vi "Teleop.vi"(10 "Match Info":T1={"Autonomous Elapsed Seconds"=0.0, "TeleOp Elapsed Seconds"=0.0, "Disabled Elapsed Seconds"=0.0, "Visited Autonomous"=FALSE, "Visited TeleOp"=FALSE, "Visited Disabled"=FALSE, "Autonomous Settings"={"Autonomous Style"=enum."Independent", "VI Refnum"=refnum}}, 11 "Call Context":T2) -> ()   [LabVIEW 2014]
doc: "This VI is called for each TeleOp packet received from the DS where the robot is not disabled. It is often used to read from the joysticks and update I/O or to update setpoints for timed control loops. It should complete and return within 20 milliseconds or it may miss DS packets."
uses:
  <vilib>/Rock Robotics/WPI/DriverStation/WPI_DriverStationDerivedRobotMode.ctl
  <vilib>/Rock Robotics/WPI/DriverStation/WPI_DriverStationMatch Info.ctl
  <vilib>/Rock Robotics/WPI/Joystick/WPI_JoystickGetSetRefNum.vi
  Robot Global Data.vi
panel:
  out "Loop Time":cluster{"X":dbl[], "Y":dbl[]}(graph)
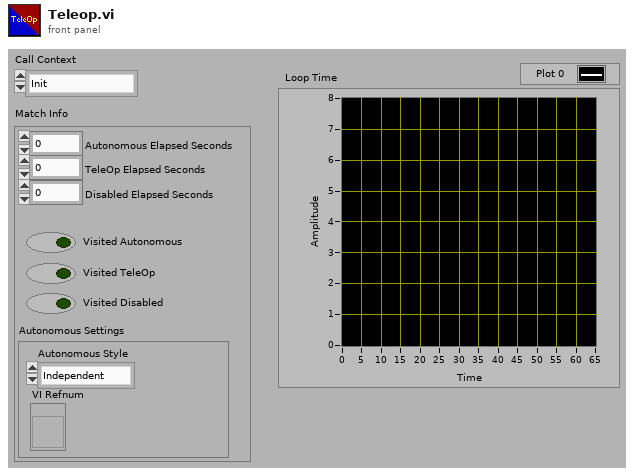
[diagram p1: front panel]
types:
  T1 = typedef "WPI_DriverStationMatch Info.ctl" = cluster{"Autonomous Elapsed Seconds":dbl, "TeleOp Elapsed Seconds":dbl, "Disabled Elapsed Seconds":dbl, "Visited Autonomous":bool, "Visited TeleOp":bool, "Visited Disabled":bool, "Autonomous Settings":cluster{"Autonomous Style":enum16{"Iterative", "Independent"}, "VI Refnum":refnum<vi>}}
  T2 = typedef "WPI_DriverStationDerivedRobotMode.ctl" = enum16{"Init", "Execute", "Stop"}
  T3 = typedef "WPI_JoystickDevRef.ctl" = cluster{"Device":T4}
  T4 = typedef "WPI_JoystickDeviceEnum.ctl" = enum16{"USB 0", "USB 1", "USB 2", "USB 3", "USB 4", "USB 5"}
  T5 = cluster{"Motor Speed":dbl, "Grabber":bool, "Go Up a Level":bool, "Go Down a Level":bool}
  T6 = cluster{"Lifter Down":bool, "Right Infeed":enum16{"Off", "Forward", "Reverse"}, "Left Infeed":enum16{"Off", "Forward", "Reverse"}}
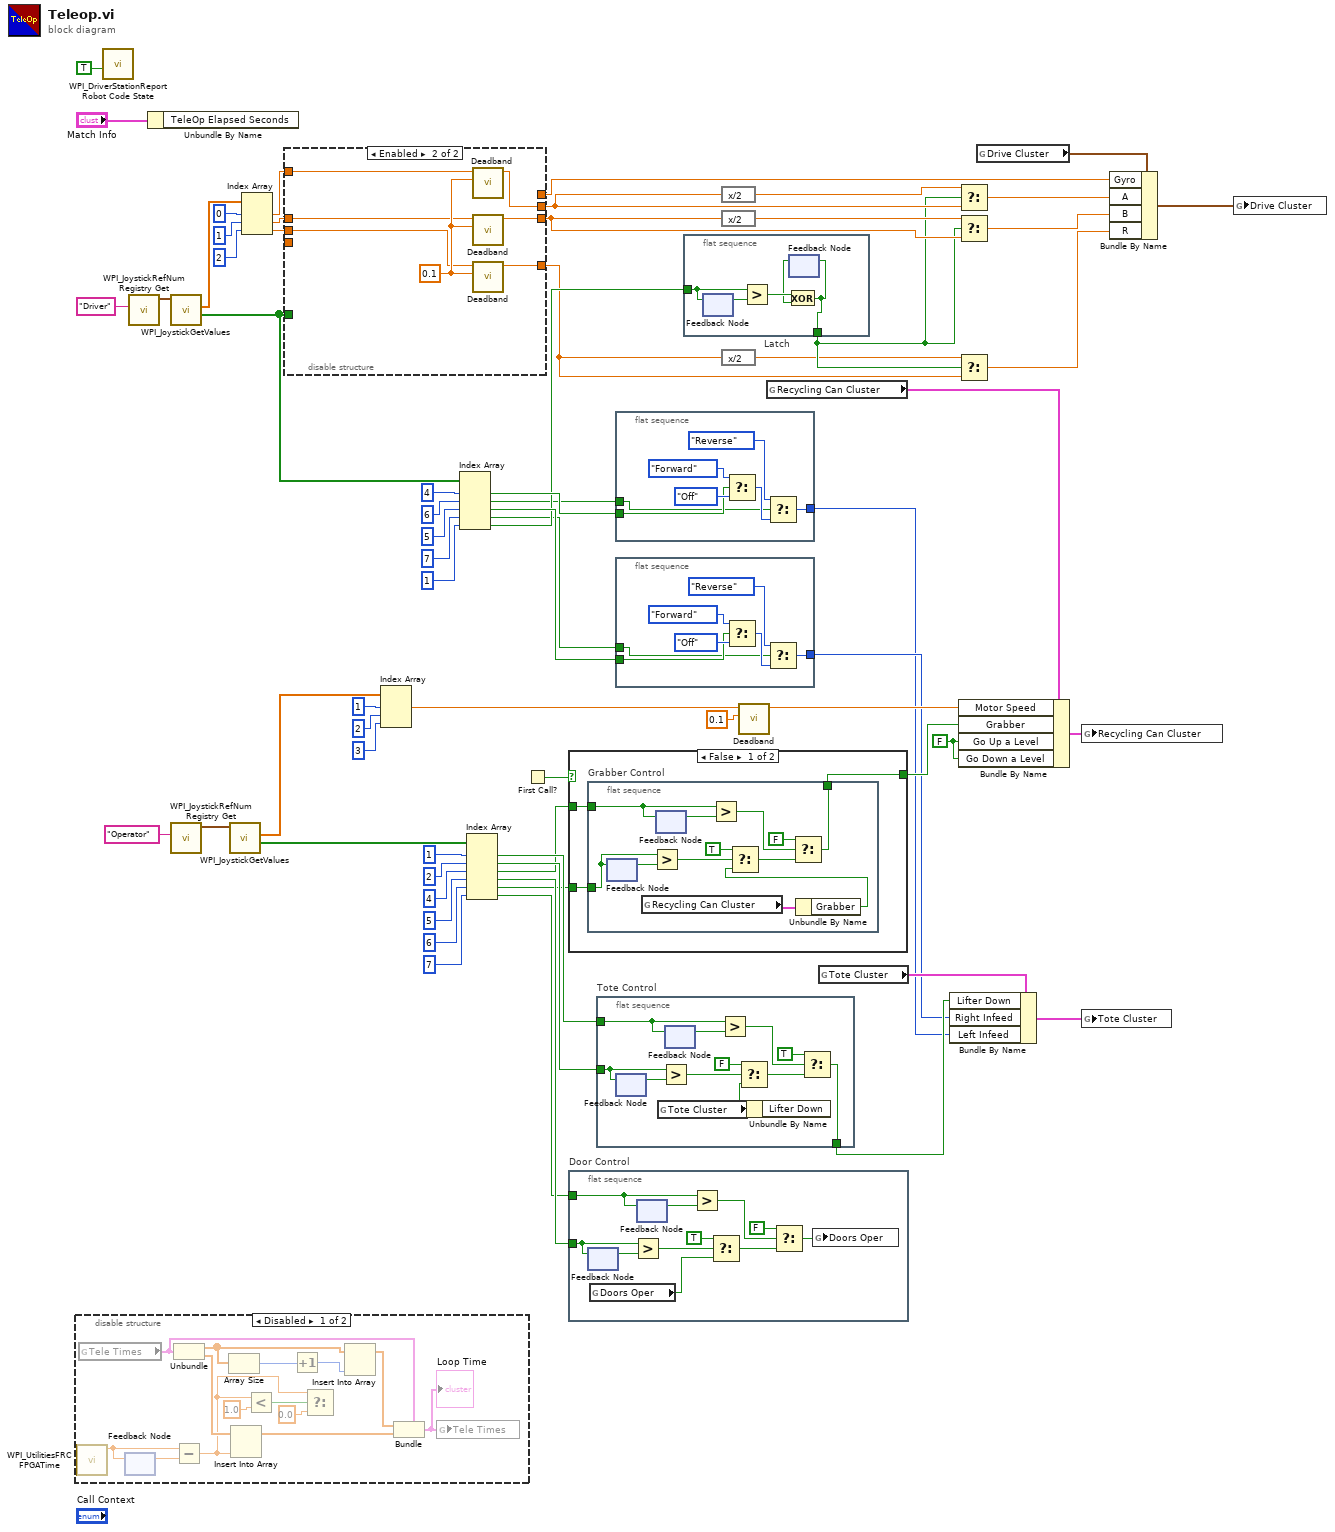
[diagram p0: block diagram]
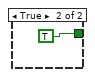
[diagram p3: hidden frame]
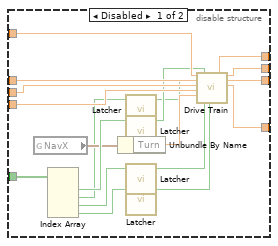
[diagram p4: hidden frame]
diagram:
  w28 = FALSE ("Go Up a Level")
  n1 = disable-structure shown="Disabled" {
    frame Disabled {
      n2 = call <vilib>:"WPI_UtilitiesFRC FPGATime.vi"() -> ("FPGA Time"=w68:dbl)  [unwired: 10 in, 1 out]
      n3 = global read "Robot Global Data.vi" "Tele Times"() -> (w81:cluster{"X":dbl[], "Y":dbl[]})
      n4 = feedback #1() -> (w74:dbl)  [unwired: 1 in]
      n5 = feedback-in #1(w68) -> ()
      n6 = Unbundle(w81) -> ("X"=w79:dbl[], "Y"=w76:dbl[])
      n7 = Subtract(x=w68, y=w74) -> (x-y=w69:dbl)
      n8 = Array Size(array=w79) -> (size(s)=w80:i32)
      n9 = Insert Into Array(array=w76, new element=w69) -> (w75:dbl[])  [unwired: 1 in]
      n10 = Less?(x=w69, y=1.0) -> (x < y?=w71:bool)
      n11 = Increment(x=w80) -> (x+1=w78:i32)
      n12 = Select(t=w69, s=w71, f=0.0 ("t")) -> ()  [unwired: 1 out]
      n13 = Insert Into Array(array=w79, new element=w78) -> (w77:dbl[])  [unwired: 1 in]
      n14 = Bundle(cluster=w81, "X"=w77, "Y"=w75) -> (w73:cluster{"X":dbl[], "Y":dbl[]})
      "Loop Time" <- w73
      n15 = global write "Robot Global Data.vi" "Tele Times"(w73) -> ()
    }
    frame Enabled {
    }
  }
  n16 = call <vilib>:"WPI_DriverStationReport Robot Code State.vi"("TeleOp"=TRUE ("Autonomous")) -> ()  [unwired: 10 in, 1 out]
  n17 = call <vilib>:"WPI_JoystickRefNum Registry Get.vi"("refnum name"="Driver") -> ("JoystickDevRef"=w64:T3)  [unwired: 9 in, 1 out]
  n18 = Unbundle By Name("Match Info") -> ()  [unwired: 1 out]
  n19 = call <vilib>:"WPI_JoystickGetValues.vi"("JoystickDevRef"=w64) -> ("Buttons"=w45:bool[], "Axes"=w47:dbl[])  [unwired: 6 in, 3 out]
  n20 = call <vilib>:"WPI_JoystickRefNum Registry Get.vi"("refnum name"="Operator") -> ("JoystickDevRef"=w53:T3)  [unwired: 9 in, 1 out]
  n21 = call <vilib>:"WPI_JoystickGetValues.vi"("JoystickDevRef"=w53) -> ("Buttons"=w38:bool[], "Axes"=w48:dbl[])  [unwired: 6 in, 3 out]
  n22 = Index Array(array=w47, index #1=0 ("index"), index #2=1 ("index"), index #3=2 ("index")) -> (element #1=w61:dbl, element #2=w60:dbl, element #3=w59:dbl)
  n23 = disable-structure shown="Enabled" {
    disable-tunnel: [w100 w107] -> w16
    disable-tunnel: [w99 w105] -> w17
    disable-tunnel: [w98 w104] -> w8
    disable-tunnel: w45 -> [w97 _]
    disable-tunnel: w61 -> [w89 w103]
    disable-tunnel: w60 -> [w88 w102]
    disable-tunnel: w59 -> [w87 w101]
    disable-tunnel: _ -> [w86 _]
    disable-tunnel: [w85 _] -> w58
    frame Disabled {
      n24 = global read "Robot Global Data.vi" "NavX"() -> (w91:cluster{"Update Speed (Hz)":dbl, "Turn":dbl})
      n25 = Index Array(array=w97) -> (element #1=w96:bool, element #2=w83:bool, element #3=w95:bool, element #4=w94:bool)  [unwired: 4 in]
      n26 = Unbundle By Name(w91) -> ("Turn"=w90:dbl)
      n27 = call "Latcher.vi"("Value In"=w83) -> ("Latched"=w82:bool)  [unwired: 4 in]
      n28 = call "Latcher.vi"("Value In"=w96) -> ("Latched"=w84:bool)  [unwired: 4 in]
      n29 = call "Latcher.vi"("Value In"=w95) -> ("Latched"=w92:bool)  [unwired: 4 in]
      n30 = call "Latcher.vi"("Value In"=w94) -> ("Latched"=w93:bool)  [unwired: 4 in]
      n31 = call "Drive Train.vi"("C"=w89, "D"=w88, "X"=w87, "Y"=w86, "gyro"=w90, "Mode Switch"=w84, "Positive 1"=w92, 8:w82, "Negative 1"=w93) -> ("gyro angle"=w85:dbl, "A"=w100:dbl, "B"=w99:dbl, "R"=w98:dbl)  [unwired: 7 in]
    }
    frame Enabled {
      w106 = 0.1 ("y")
      n32 = call "Deadband.vi"("Deadband"=w106, "Motor Speed"=w103) -> ("Power Out"=w107:dbl)  [unwired: 9 in]
      n33 = call "Deadband.vi"("Deadband"=w106, "Motor Speed"=w102) -> ("Power Out"=w105:dbl)  [unwired: 9 in]
      n34 = call "Deadband.vi"("Deadband"=w106, "Motor Speed"=w101) -> ("Power Out"=w104:dbl)  [unwired: 9 in]
    }
  }
  n35 = Index Array(array=w48, index #1=1 ("index"), index #2=2 ("index"), index #3=3 ("index")) -> (element #1=w26:dbl)  [unwired: 2 out]
  n36 = Index Array(array=w45, index #1=4 ("index"), index #2=6 ("index"), index #3=5 ("index"), index #4=7 ("index"), index #5=1 ("index")) -> (element #1=w39:bool, element #2=w4:bool, element #3=w40:bool, element #4=w5:bool, element #5=w12:bool)
  n37 = Index Array(array=w38, index #1=1 ("index"), index #2=2 ("index"), index #3=4 ("index"), index #4=5 ("index"), index #5=6 ("index"), index #6=7 ("index")) -> (element #1=w31:bool, element #2=w30:bool, element #3=w21:bool, element #4=w3:bool, element #5=w1:bool, element #6=w2:bool)
  n38 = First Call?() -> (First Call?: T/F=w22:bool)
  n39 = case shown="False" w22 {
    tunnel: w21 -> [w110 _]
    tunnel: w1 -> [w109 _]
    tunnel: [w108 TRUE] -> w20
    frame False {
      n40 = flat-sequence "Grabber Control" {
        tunnel: w110 -> [w118]
        tunnel: w109 -> [w114]
        tunnel: [w111] -> w108
        frame #0 {
          n41 = feedback-in #2(w114) -> ()
          n42 = feedback #2() -> (w122:bool)  [unwired: 1 in]
          n43 = global read "Robot Global Data.vi" "Recycling Can Cluster"() -> (w113:T5)
          n44 = Greater?(x=w114, y=w122) -> (0:w121:bool)
          n45 = feedback #3() -> (w119:bool)  [unwired: 1 in]
          n46 = feedback-in #3(w118) -> ()
          n47 = Greater?(x=w118, y=w119) -> (0:w117:bool)
          n48 = Unbundle By Name(w113) -> ("Grabber"=w112:bool)
          n49 = Select(t=TRUE, s=w121, f=w112) -> (s? t:f=w116:bool)
          n50 = Select(t=FALSE, s=w117, f=w116) -> (s? t:f=w111:bool)
        }
      }
    }
    frame True {
    }
  }
  n51 = flat-sequence "Door Control" {
    tunnel: w3 -> [w133]
    tunnel: w2 -> [w128]
    frame #0 {
      n52 = feedback-in #4(w133) -> ()
      n53 = feedback #4() -> (w134:bool)  [unwired: 1 in]
      n54 = global read "Robot Global Data.vi" "Doors Oper"() -> (w130:bool)
      n55 = Greater?(x=w133, y=w134) -> (0:w132:bool)
      n56 = feedback #5() -> (w129:bool)  [unwired: 1 in]
      n57 = feedback-in #5(w128) -> ()
      n58 = Greater?(x=w128, y=w129) -> (0:w127:bool)
      n59 = Select(t=TRUE, s=w132, f=w130) -> (s? t:f=w126:bool)
      n60 = Select(t=FALSE, s=w127, f=w126) -> (s? t:f=w124:bool)
      n61 = global write "Robot Global Data.vi" "Doors Oper"(w124) -> ()
    }
  }
  n62 = flat-sequence "Tote Control" {
    tunnel: w30 -> [w145]
    tunnel: w31 -> [w141]
    tunnel: [w137] -> w29
    frame #0 {
      n63 = feedback-in #6(w145) -> ()
      n64 = feedback #6() -> (w146:bool)  [unwired: 1 in]
      n65 = global read "Robot Global Data.vi" "Tote Cluster"() -> (w136:T6)
      n66 = Greater?(x=w145, y=w146) -> (0:w144:bool)
      n67 = feedback #7() -> (w142:bool)  [unwired: 1 in]
      n68 = feedback-in #7(w141) -> ()
      n69 = Greater?(x=w141, y=w142) -> (0:w140:bool)
      n70 = Unbundle By Name(w136) -> ("Lifter Down"=w135:bool)
      n71 = Select(t=FALSE, s=w144, f=w135) -> (s? t:f=w139:bool)
      n72 = Select(t=TRUE, s=w140, f=w139) -> (s? t:f=w137:bool)
    }
  }
  n73 = flat-sequence {
    tunnel: [w149] -> w6
    tunnel: w39 -> [w148]
    tunnel: w4 -> [w147]
    frame #0 {
      n74 = Select(t=enum16{"Off", "Forward", "Reverse"}."Forward" ("Right Infeed"), s=w148, f=enum16{"Off", "Forward", "Reverse"}."Off" ("Right Infeed")) -> (s? t:f=w153:enum16{"Off", "Forward", "Reverse"})
      n75 = Select(t=enum16{"Off", "Forward", "Reverse"}."Reverse" ("Right Infeed"), s=w147, f=w153) -> (s? t:f=w149:enum16{"Off", "Forward", "Reverse"})
    }
  }
  n76 = flat-sequence {
    tunnel: w40 -> [w156]
    tunnel: w5 -> [w155]
    tunnel: [w154] -> w7
    frame #0 {
      n77 = Select(t=enum16{"Off", "Forward", "Reverse"}."Forward" ("Right Infeed"), s=w156, f=enum16{"Off", "Forward", "Reverse"}."Off" ("Right Infeed")) -> (s? t:f=w160:enum16{"Off", "Forward", "Reverse"})
      n78 = Select(t=enum16{"Off", "Forward", "Reverse"}."Reverse" ("Right Infeed"), s=w155, f=w160) -> (s? t:f=w154:enum16{"Off", "Forward", "Reverse"})
    }
  }
  n79 = flat-sequence "Latch" {
    tunnel: w12 -> [w162]
    tunnel: [w161] -> w11
    frame #0 {
      n80 = feedback #8() -> (w163:bool)  [unwired: 1 in]
      n81 = feedback-in #8(w162) -> ()
      n82 = Greater?(x=w162, y=w163) -> (0:w165:bool)
      n83 = feedback #9() -> (w164:bool)  [unwired: 1 in]
      n84 = Exclusive Or(1:w164, 2:w165) -> (0:w161:bool)
      n85 = feedback-in #9(w161) -> ()
    }
  }
  n86 = expression code="x/2"(w16) -> (w19:dbl)
  n87 = expression code="x/2"(w17) -> (w18:dbl)
  n88 = expression code="x/2"(w8) -> (w9:dbl)
  n89 = call "Deadband.vi"("Deadband"=0.1, "Motor Speed"=w26) -> ("Power Out"=w25:dbl)  [unwired: 9 in]
  n90 = global read "Robot Global Data.vi" "Recycling Can Cluster"() -> (w52:T5)
  n91 = global read "Robot Global Data.vi" "Tote Cluster"() -> (w50:T6)
  n92 = Bundle By Name(cluster=w50, "Lifter Down"=w29, "Right Infeed"=w7, "Left Infeed"=w6) -> (w49:T6)
  n93 = Select(t=w19, s=w11, f=w16) -> (s? t:f=w14:dbl)
  n94 = Select(t=w18, s=w11, f=w17) -> (s? t:f=w15:dbl)
  n95 = Select(t=w9, s=w11, f=w8) -> (s? t:f=w10:dbl)
  n96 = Bundle By Name(cluster=w52, "Motor Speed"=w25, "Grabber"=w20, "Go Up a Level"=w28, "Go Down a Level"=w28) -> (w51:T5)
  n97 = global read "Robot Global Data.vi" "Drive Cluster"() -> (w63:cluster{"A":dbl, "B":dbl, "R":dbl, "Gyro":dbl})
  n98 = global write "Robot Global Data.vi" "Recycling Can Cluster"(w51) -> ()
  n99 = global write "Robot Global Data.vi" "Tote Cluster"(w49) -> ()
  n100 = Bundle By Name(cluster=w63, "Gyro"=w58, "A"=w14, "B"=w15, "R"=w10) -> (w62:cluster{"A":dbl, "B":dbl, "R":dbl, "Gyro":dbl})
  n101 = global write "Robot Global Data.vi" "Drive Cluster"(w62) -> ()
